vi "Call the Error VI Creator by Reference.vi"(8 "error in":errorcluster, 9 "Calling mode":T1, 11 "Selection":T2) -> (0 "error out":errorcluster, 1 "Error VI Path":path, 2 "Cancel Out":bool)   [LabVIEW 2020, in "Panther Dashboard.lvlib"]
uses:
  Panther Dashboard.lvlib
  <vilib>/PantherLAB/Panther Constants and Errors/Libraries/ConstantErrorsMaker/Selection Info--cluster.ctl
  <vilib>/PantherLAB/Panther Constants and Errors/Libraries/ConstantErrorsMaker/Selection Type--enum.ctl
  Calling mode--enum.ctl
  <vilib>/PantherLAB/Panther Constants and Errors/Libraries/ConstantErrorsMaker/PantherLAB_lib_ConstantErrorsMaker.lvlib
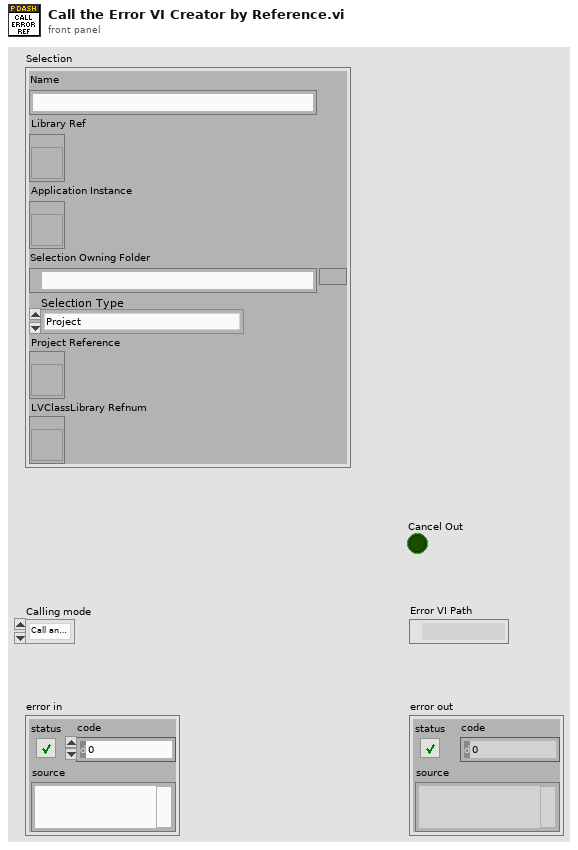
[diagram p1: front panel]
types:
  T1 = typedef "Panther Dashboard.lvlib/Calling mode--enum.ctl" = enum16{"Call and Forguet", "Call and Collect"}
  T2 = typedef "PantherLAB_lib_ConstantErrorsMaker.lvlib/Selection Info--cluster.ctl" = cluster{"Name":string, "Library Ref":refnum<vi>, "Application Instance":refnum<vi>, "Selection Owning Folder":path, "Selection Type":T3, "Project Reference":refnum<vi>, "LVClassLibrary Refnum":refnum<vi>}
  T3 = typedef "PantherLAB_lib_ConstantErrorsMaker.lvlib/Selection Type--enum.ctl" = enum16{"Project", "Library", "Class", "DQMH Singleton", "DQMH Cloneable"}
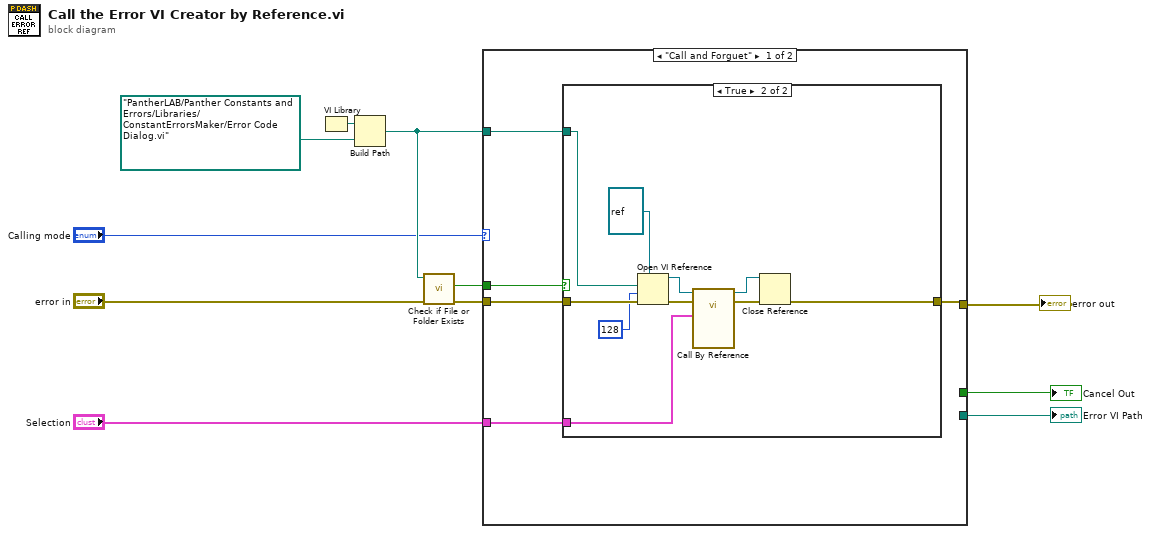
[diagram p0: block diagram]
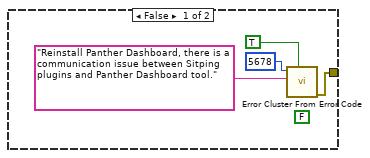
[diagram p2: hidden frame]
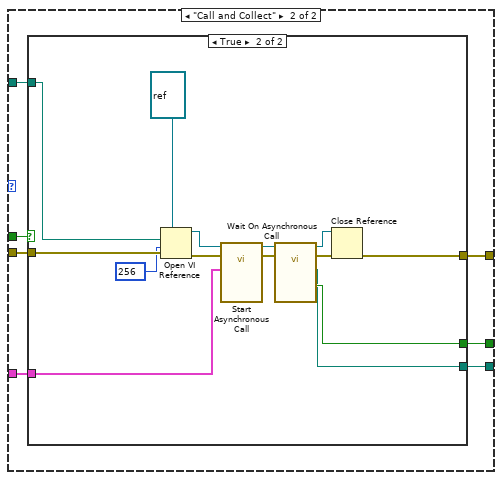
[diagram p3: hidden frame]
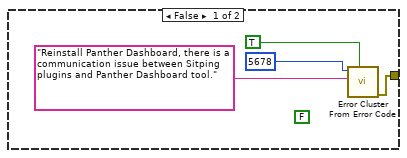
[diagram p4: hidden frame]
diagram:
  n1 = VI Library() -> (path=w4:path)
  n2 = Build Path(base path=w4, name or relative path=path "PantherLAB/Panther Constants and Errors/Libraries/ConstantErrorsMaker/Error Code Dialog.vi") -> (appended path=w7:path)
  n3 = call <vilib>:"Check if File or Folder Exists.vi"("error in (no error)"="error in", "path"=w7) -> ("error out"=w9:errorcluster, "file or folder exists?"=w6:bool)  [unwired: 7 in, 1 out]
  n4 = case shown="\"Call and Forguet\"" "Calling mode" {
    tunnel: "Selection" -> [w14 w35]
    tunnel: w7 -> [w13 w34]
    tunnel: w6 -> [w12 w33]
    tunnel: [w16 w37] -> w10
    tunnel: w9 -> [w15 w36]
    tunnel: [_ w32] -> w2
    tunnel: [_ w31] -> w1
    frame "Call and Forguet" {
      n5 = case shown="True" w12 {
        tunnel: w15 -> [_ w28]
        tunnel: w13 -> [_ w24]
        tunnel: [w20 w27] -> w16
        tunnel: w14 -> [_ w22]
        frame False {
          (unwired) FALSE
          n6 = call <vilib>:"Error Cluster From Error Code.vi"("show call chain? (False)"=TRUE, "error message (\"\")"="Reinstall Panther Dashboard, there is a communication issue between Sitping plugins and Panther Dashboard tool." ("error message (\"\")"), "error code (0)"=5678) -> ("error out"=w20:errorcluster)  [unwired: 6 in]
        }
        frame True {
          n7 = Open VI Reference(type specifier VI Refnum (for type only)=refnum<vi> refnum, vi path=w24, options=128, error in (no error)=w28) -> (vi reference=w25:refnum<vi>, error out=w29:errorcluster)  [unwired: 2 in]
          n8 = call-by-ref "?"(reference=w25, error in=w29, "Selection"=w22) -> (reference out=w26:refnum<vi>, error out=w30:errorcluster)  [unwired: 8 in, 3 out]
          n9 = Close Reference(reference=w26, error in (no error)=w30) -> (error out=w27:errorcluster)
        }
      }
    }
    frame "Call and Collect" {
      n10 = case shown="True" w33 {
        tunnel: w36 -> [_ w55]
        tunnel: w34 -> [_ w50]
        tunnel: [w41 w54] -> w37
        tunnel: w35 -> [_ w46]
        tunnel: [_ w43] -> w32
        tunnel: [_ w42] -> w31
        frame False {
          (unwired) FALSE
          n11 = call <vilib>:"Error Cluster From Error Code.vi"("show call chain? (False)"=TRUE, "error message (\"\")"="Reinstall Panther Dashboard, there is a communication issue between Sitping plugins and Panther Dashboard tool." ("error message (\"\")"), "error code (0)"=5678) -> ("error out"=w41:errorcluster)  [unwired: 6 in]
        }
        frame True {
          n12 = Open VI Reference(type specifier VI Refnum (for type only)=refnum<vi> refnum, vi path=w50, options=256, error in (no error)=w55) -> (vi reference=w47:refnum<vi>, error out=w53:errorcluster)  [unwired: 2 in]
          n13 = call-by-ref "Start Asynchronous Call"(reference=w47, error in=w53, "Selection"=w46) -> (reference out=w45:refnum<vi>, error out=w51:errorcluster)  [unwired: 8 in, 3 out]
          n14 = call-by-ref "Wait On Asynchronous Call"(reference=w45, error in=w51) -> (reference out=w44:refnum<vi>, error out=w52:errorcluster, "Cancel Out"=w43:bool, "Error VI Path"=w42:path)  [unwired: 9 in, 1 out]
          n15 = Close Reference(reference=w44, error in (no error)=w52) -> (error out=w54:errorcluster)
        }
      }
    }
  }
  "error out" <- w10
  "Cancel Out" <- w2
  "Error VI Path" <- w1
